vi "Proportional Control.vi"(2 "Invert?":bool, 3 "Output Range":cluster{"Lower":dbl, "Upper":dbl}, 4 "Gain":dbl, 5 "Process Variable":dbl, 6 "Setpoint":dbl) -> (0 "Output":dbl)   [LabVIEW 2013]
doc: "A proportional feedback loop. Great for controlling stuff like the temperature of Crystal's house (which by the way needs re-zoning, but not right now). This loop accomplishes the same thing as a PID if your integral and derivative gains are 0.\n\nProcess Variable is where the thing is right now, Setpoint is where you want it to be, and Gain is an arbitrary multiplier of the speed. The output speed is proportional to the difference between Process Variable and Setpoint, meaning the rate of change of your variable will decrease as the you approach your target.\n\nOutput Range allows you to limit the rate of change. By default, the range is [-100, 100]. If the loop seems to be going backwards, i.e. making the difference bigger instead of smaller, set Invert? to true."
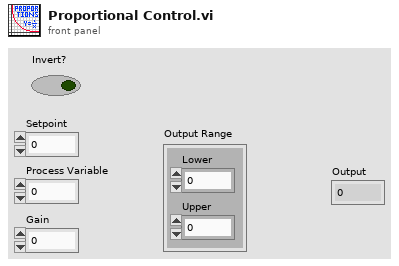
[diagram p1: front panel]
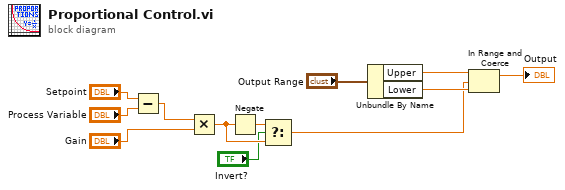
[diagram p0: block diagram]
diagram:
  n1 = Subtract(x="Setpoint", y="Process Variable") -> (x-y=w9:dbl)
  n2 = Multiply(x=w9, y="Gain") -> (x*y=w6:dbl)
  n3 = Negate(x=w6) -> (-x=w3:dbl)
  n4 = Select(t=w3, s="Invert?", f=w6) -> (s? t:f=w5:dbl)
  n5 = Unbundle By Name("Output Range") -> ("Upper"=w11:dbl, "Lower"=w10:dbl)
  n6 = In Range and Coerce(upper limit=w11, x=w5, lower limit=w10) -> (coerced(x)=→"Output":dbl)  [unwired: 1 out]
